vi "Set Voltage.vi"(8 "error in (no error)":errorcluster, 10 "Voltage (V)":dbl, 11 "Power Supply Parent in":refnum<class "Power Supply Parent.lvclass">) -> (0 "error out":errorcluster, 3 "Power Supply Parent out":refnum<class "Power Supply Parent.lvclass">)   [LabVIEW 2017, in "Power Supply Driver.lvlib" / "Power Supply Parent.lvclass"]
uses:
  Power Supply Parent.lvclass
  <vilib>/Utility/error.llb/Error Cluster From Error Code.vi
  <vilib>/ErrorRing/Error Ring.xnode
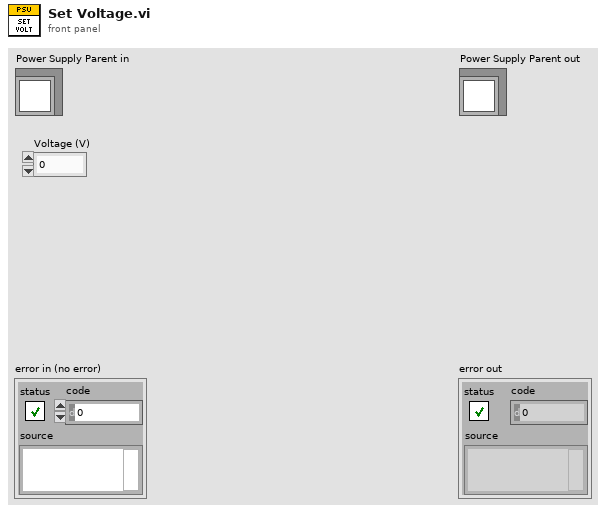
[diagram p1: front panel]
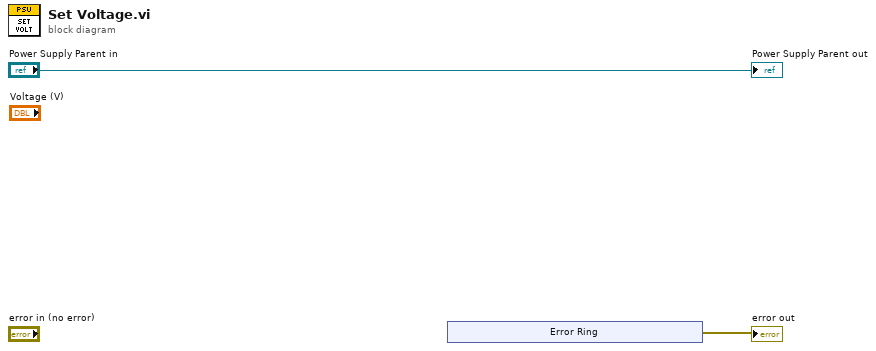
[diagram p0: block diagram]
diagram:
  n1 = xnode "Error Ring"() -> ("error out"=→"error out":errorcluster)
  "Power Supply Parent out" <- "Power Supply Parent in"
